vi "onComputeIntervals.vi"(8 "error in (no error)":errorcluster, 9 "Cron Interval":T1, 10 "Expression":string, 11 "Cron.Jenkins in":refnum<class "Cron.Jenkins.lvclass">) -> (0 "error out":errorcluster, 2 "Interval Parameters":T2, 3 "Cron.Jenkins out":refnum<class "Cron.Jenkins.lvclass">)   [LabVIEW 2013, in "openCron.lvlib" / "Cron.Jenkins.lvclass"]
uses:
  Cron.Jenkins.lvclass
  Cron/Cron Interval -- cluster.ctl
  Cron/Cron Interval -- enum.ctl
  Cron.Jenkins.lvclass/Cron.Jenkins.ctl
  <vilib>/Utility/MD5Checksum.llb/MD5Checksum string.vi
  Cron/Cron.lvclass
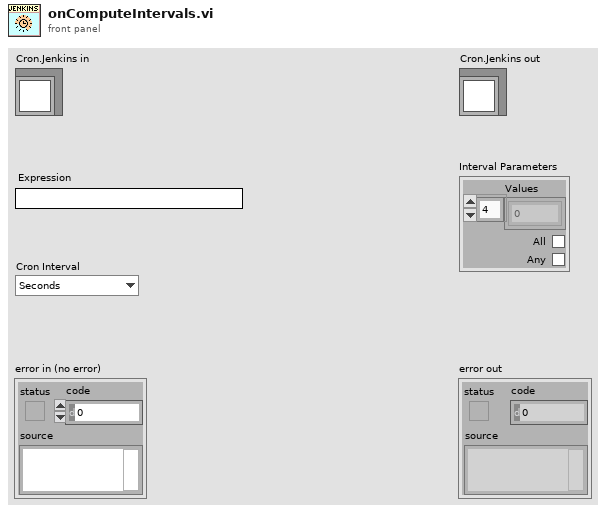
[diagram p1: front panel]
types:
  T1 = typedef "openCron.lvlib/Cron.lvclass/Cron Interval -- enum.ctl" = enum16{"Seconds", "Minutes", "Hours", "Day of Month", "Month", "Day of Week", "Year"}
  T2 = typedef "openCron.lvlib/Cron.lvclass/Cron Interval -- cluster.ctl" = cluster{"Values":i32[], "All":bool, "Any":bool}
  T3 = enum16{"SUN", "MON", "TUE", "WED", "THU", "FRI", "SAT"}
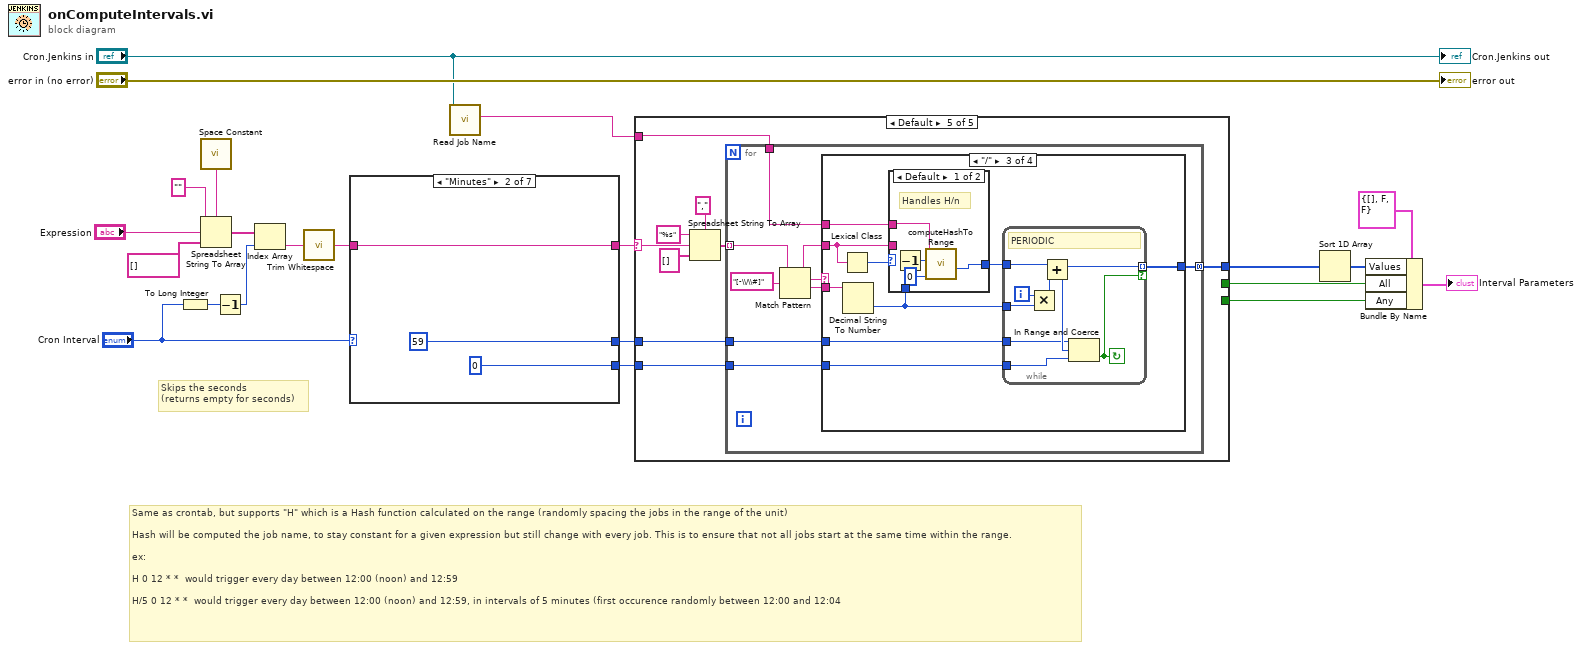
[diagram p0: block diagram]
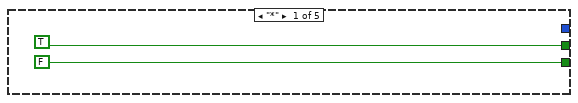
[diagram p2: hidden frame]
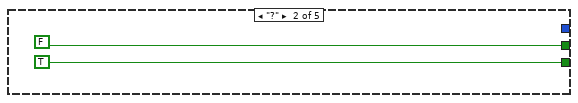
[diagram p3: hidden frame]
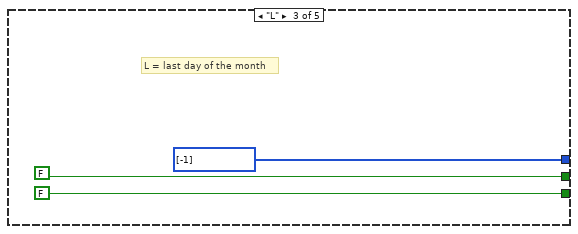
[diagram p4: hidden frame]
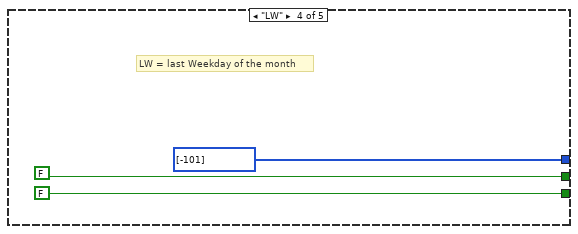
[diagram p5: hidden frame]
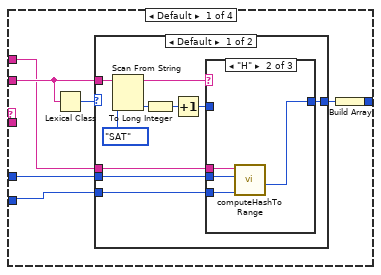
[diagram p6: hidden frame]
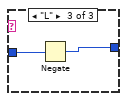
[diagram p8: hidden frame]
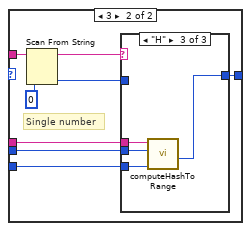
[diagram p9: hidden frame]
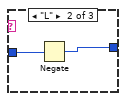
[diagram p11: hidden frame]
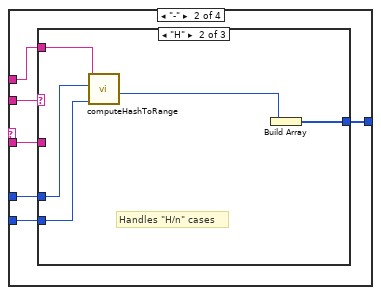
[diagram p12: hidden frame]
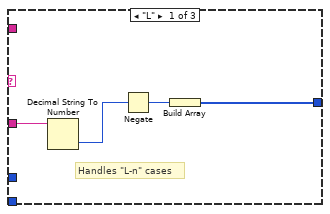
[diagram p13: hidden frame]
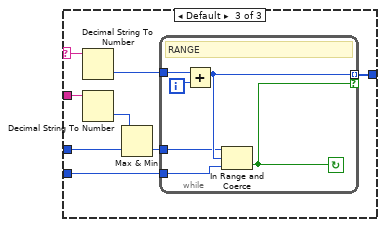
[diagram p14: hidden frame]
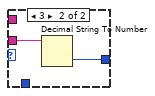
[diagram p15: hidden frame]
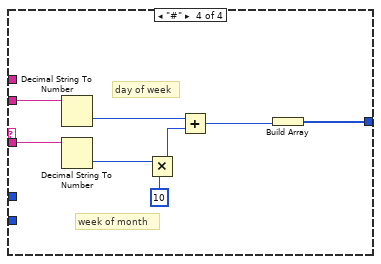
[diagram p16: hidden frame]
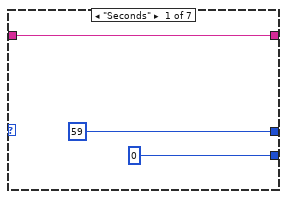
[diagram p17: hidden frame]
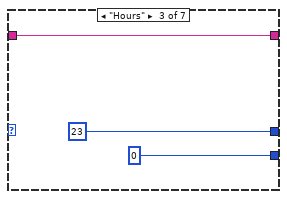
[diagram p18: hidden frame]
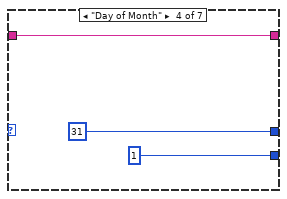
[diagram p19: hidden frame]
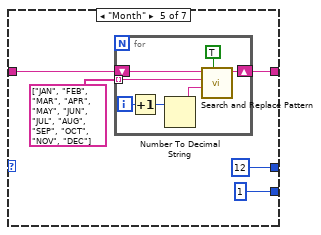
[diagram p20: hidden frame]
diagram:
  # "Skips the seconds\n(returns empty for seconds)"
  # "Same as crontab, but supports \"H\" which is a Hash function calculated on the range (randomly spacing the jobs in the range of the unit)\n\nHash will be computed the job name, to stay constant for a given expression but still change with every job. This is to ensure that not all jobs start at the same time within the range.\n\nex: \n\nH 0 12 * *  would trigger every day between 12:00 (noon) and 12:59\n \nH/5 0 12 * *  would trigger every day between 12:00 (noon) and 12:59, in intervals of 5 minutes (first occurence randomly between 12:00 and 12:04"
  n1 = To Long Integer(number="Cron Interval") -> (32bit integer=w5:i32)
  n2 = call <vilib>:"Space Constant.vi"() -> ("String"=w18:string)
  n3 = Spreadsheet String To Array(delimiter (Tab)=w18, format string="", spreadsheet string="Expression", array type (2D Dbl)=string[] []) -> (array=w17:string[])
  n4 = Decrement(x=w5) -> (x-1=w3:i32)
  n5 = Index Array(array=w17, index=w3) -> (element=w15:string)
  n6 = call <vilib>:"Trim Whitespace.vi"("string"=w15) -> ("trimmed string"=w7:string)  [unwired: 1 in]
  n7 = case shown="\"Minutes\"" "Cron Interval" {
    tunnel: [59 ("y") 59 ("y") 23 ("y") 31 ("y") 12 ("y") 7 ("y") 2099 ("y")] -> w14
    tunnel: [0 ("y") 0 ("y") 0 ("y") 1 ("y") 1 ("y") 1 ("y") 1970 ("y")] -> w13
    tunnel: w7 -> [w23 w26 w29 w32 w36 w48 w58]
    tunnel: [w23 w26 w29 w32 w37 w47 w58] -> w6
    frame "Seconds" {
    }
    frame "Minutes" {
    }
    frame "Hours" {
    }
    frame "Day of Month" {
    }
    frame "Month" {
      n8 = for {
        shift-right: [w46] -> w37
        shift-left: w36 -> [w45]
        tunnel: string[] ["JAN", "FEB", "MAR", "APR", "MAY", "JUN", "JUL", "AUG", "SEP", "OCT", "NOV", "DEC"] -> [w43] mode=indexing
        i -> [w42]
        n9 = Increment(x=w42) -> (x+1=w41:i32)
        n10 = Number To Decimal String(number=w41) -> (decimal integer string=w40:string)  [unwired: 1 in]
        n11 = call <vilib>:"Search and Replace Pattern.vi"("string"=w45, "regular expression (\"\")"=w43, "replace string (\"\")"=w40, "replace all? (F)"=TRUE) -> ("result string"=w46:string)  [unwired: 1 in, 1 out]
      }
    }
    frame "Day of Week" {
      n12 = for {
        shift-right: [w57] -> w47
        shift-left: w48 -> [w56]
        tunnel: string[] ["SUN", "MON", "TUE", "WED", "THU", "FRI", "SAT"] -> [w54] mode=indexing
        i -> [w52]
        n13 = Number To Decimal String(number=w52) -> (decimal integer string=w53:string)  [unwired: 1 in]
        n14 = call <vilib>:"Search and Replace Pattern.vi"("string"=w56, "regular expression (\"\")"=w54, "replace string (\"\")"=w53, "replace all? (F)"=TRUE) -> ("result string"=w57:string)  [unwired: 1 in, 1 out]
      }
    }
    frame "Year" {
    }
  }
  n15 = call "Read Job Name.vi"("Cron.Jenkins in"="Cron.Jenkins in") -> ("Job Name"=w1:string)  [unwired: 8 in, 2 out]
  n16 = case shown="Default" w6 {
    selector: w6 -> [_ _ _ _ w75]
    tunnel: [_ _ i32[] [-1] i32[] [-101] w74] -> w11
    tunnel: [TRUE FALSE FALSE FALSE _] -> w10
    tunnel: [FALSE TRUE FALSE FALSE _] -> w9
    tunnel: w14 -> [_ _ _ _ w73]
    tunnel: w13 -> [_ _ _ _ w72]
    tunnel: w1 -> [_ _ _ _ w71]
    frame "*" {
    }
    frame "?" {
    }
    frame "L" {
      # "L = last day of the month"
    }
    frame "LW" {
      # "LW = last Weekday of the month"
    }
    frame Default {
      n17 = Spreadsheet String To Array(delimiter (Tab)=",", format string="%s", spreadsheet string=w75, array type (2D Dbl)=string[] []) -> (array=w76:string[])
      n18 = for {
        tunnel: w76 -> [w88] mode=indexing
        tunnel: [w84] -> w74 mode=concatenating
        tunnel: w73 -> [w82]
        tunnel: w72 -> [w81]
        tunnel: w71 -> [w80]
        n19 = Match Pattern(string=w88, regular expression="[-\\/\\#]") -> (before substring=w85:string, match substring=w86:string, after substring=w83:string)  [unwired: 1 in, 1 out]
        n20 = case shown="\"/\"" w86 {
          tunnel: w85 -> [w93 w129 w160 w188]
          tunnel: [w94 w132 w164 w186] -> w84
          tunnel: w83 -> [_ w133 w163 w187]
          tunnel: w82 -> [w90 w131 w162 _]
          tunnel: w81 -> [w89 w130 w161 _]
          tunnel: w80 -> [w91 w128 w158 _]
          frame Default {
            n21 = Lexical Class(1:w93) -> (0:w92:i16)
            n22 = case shown="Default" w92 {
              tunnel: [w99 w118] -> w95
              tunnel: w93 -> [w105 w120]
              tunnel: w91 -> [w98 w115]
              tunnel: w90 -> [w97 w114]
              tunnel: w89 -> [w96 w113]
              frame Default {
                n23 = Scan From String(input string=w105, default 1=T3."SAT" ("y")) -> (remaining string=w101:string, output 1=w102:T3)  [unwired: 3 in, 2 out]
                n24 = To Long Integer(number=w102) -> (32bit integer=w103:i32)
                n25 = Increment(x=w103) -> (x+1=w100:i32)
                n26 = case shown="\"H\"" w101 {
                  tunnel: w100 -> [w106 _ w112]
                  tunnel: [w106 w107 w111] -> w99
                  tunnel: w98 -> [_ w110 _]
                  tunnel: w97 -> [_ w109 _]
                  tunnel: w96 -> [_ w108 _]
                  frame Default {
                  }
                  frame "H" {
                    n27 = call "computeHashToRange.vi"("min Value"=w108, "maxValue"=w109, "seed"=w110) -> ("H"=w107:i32)  [unwired: 8 in]
                  }
                  frame "L" {
                    n28 = Negate(x=w112) -> (-x=w111:i32)
                  }
                }
              }
              frame 3 {
                # "Single number"
                n29 = Scan From String(input string=w120, default 1=0 ("32bit integer")) -> (remaining string=w119:string, output 1=w116:i32)  [unwired: 3 in, 2 out]
                n30 = case shown="\"H\"" w119 {
                  tunnel: w116 -> [w121 w123 _]
                  tunnel: [w121 w122 w124] -> w118
                  tunnel: w115 -> [_ _ w127]
                  tunnel: w114 -> [_ _ w126]
                  tunnel: w113 -> [_ _ w125]
                  frame Default {
                  }
                  frame "L" {
                    n31 = Negate(x=w123) -> (-x=w122:i32)
                  }
                  frame "H" {
                    n32 = call "computeHashToRange.vi"("min Value"=w125, "maxValue"=w126, "seed"=w127) -> ("H"=w124:i32)  [unwired: 8 in]
                  }
                }
              }
            }
            n33 = Build Array(w95) -> (w94:i32[])
          }
          frame "-" {
            n34 = case shown="\"H\"" w129 {
              selector: w129 -> [_ _ w143]
              tunnel: w133 -> [w137 _ w149]
              tunnel: [w135 w142 w148] -> w132
              tunnel: w131 -> [_ w140 w146]
              tunnel: w130 -> [_ w139 w145]
              tunnel: w128 -> [_ w141 _]
              frame "L" {
                # "Handles \"L-n\" cases"
                n35 = Decimal String To Number(string=w137) -> (number=w136:i32)  [unwired: 2 in, 1 out]
                n36 = Negate(x=w136) -> (-x=w134:i32)
                n37 = Build Array(w134) -> (w135:i32[])
              }
              frame "H" {
                # "Handles \"H/n\" cases"
                n38 = call "computeHashToRange.vi"("min Value"=w139, "maxValue"=w140, "seed"=w141) -> ("H"=w138:i32)  [unwired: 8 in]
                n39 = Build Array(w138) -> (w142:i32[])
              }
              frame Default {
                n40 = Decimal String To Number(string=w143) -> (number=w150:i32)  [unwired: 2 in, 1 out]
                n41 = Decimal String To Number(string=w149) -> (number=w147:i32)  [unwired: 2 in, 1 out]
                n42 = Max & Min(x=w147, y=w146) -> (min(x,y)=w144:i32)  [unwired: 1 out]
                n43 = while {
                  tunnel: w150 -> [w156]
                  tunnel: [w153] -> w148 mode=indexing if=w154
                  tunnel: w145 -> [w152]
                  tunnel: w144 -> [w151]
                  i -> [w155]
                  stop <- w154 continue-if-true
                  # "RANGE"
                  n44 = Add(x=w156, y=w155) -> (x+y=w153:i32)
                  n45 = In Range and Coerce(upper limit=w151, x=w153, lower limit=w152) -> (In Range?=w154:bool)  [unwired: 1 out]
                }
              }
            }
          }
          frame "/" {
            n46 = Lexical Class(1:w160) -> (0:w159:i16)
            n47 = Decimal String To Number(string=w163) -> (number=w157:i32)  [unwired: 2 in, 1 out]
            n48 = case shown="Default" w159 {
              tunnel: [w167 w172] -> w165
              tunnel: w160 -> [_ w171]
              tunnel: w158 -> [w168 _]
              tunnel: w157 -> [w170 _]
              frame Default {
                # "Handles H/n"
                n49 = Decrement(x=w170) -> (x-1=w166:i32)
                n50 = call "computeHashToRange.vi"("min Value"=0, "maxValue"=w166, "seed"=w168) -> ("H"=w167:i32)  [unwired: 8 in]
              }
              frame 3 {
                n51 = Decimal String To Number(string=w171) -> (number=w172:i32)  [unwired: 2 in, 1 out]
              }
            }
            n52 = while {
              tunnel: w165 -> [w180]
              tunnel: [w176] -> w164 mode=indexing if=w173
              tunnel: w157 -> [w179]
              tunnel: w162 -> [w175]
              tunnel: w161 -> [w174]
              i -> [w178]
              stop <- w173 continue-if-true
              # "PERIODIC"
              n53 = Multiply(x=w178, y=w179) -> (x*y=w177:i32)
              n54 = Add(x=w180, y=w177) -> (x+y=w176:i32)
              n55 = In Range and Coerce(upper limit=w175, x=w176, lower limit=w174) -> (In Range?=w173:bool)  [unwired: 1 out]
            }
          }
          frame "#" {
            # "week of month"
            # "day of week"
            n56 = Decimal String To Number(string=w188) -> (number=w183:i32)  [unwired: 2 in, 1 out]
            n57 = Decimal String To Number(string=w187) -> (number=w185:i32)  [unwired: 2 in, 1 out]
            n58 = Multiply(x=w185, y=10) -> (x*y=w182:i32)
            n59 = Add(x=w183, y=w182) -> (x+y=w181:i32)
            n60 = Build Array(w181) -> (w186:i32[])
          }
        }
      }
    }
  }
  n61 = Sort 1D Array(array=w11) -> (sorted array=w12:i32[])
  n62 = Bundle By Name(cluster=T2 {"Values"=[], "All"=FALSE, "Any"=FALSE} ("Interval"), "Values"=w12, "All"=w10, "Any"=w9) -> (→"Interval Parameters":T2)
  "error out" <- "error in (no error)"
  "Cron.Jenkins out" <- "Cron.Jenkins in"
